vi "Close.vi"(8 "error in (no error)":errorcluster, 11 "Data in":refnum<class "Local Bus.lvclass">) -> (0 "error out":errorcluster, 3 "Data out":refnum<class "Local Bus.lvclass">)   [LabVIEW 2021, in "Local Bus.lvclass"]
uses:
  Local Bus.lvclass
  Local Bus.lvclass/Local Bus.ctl
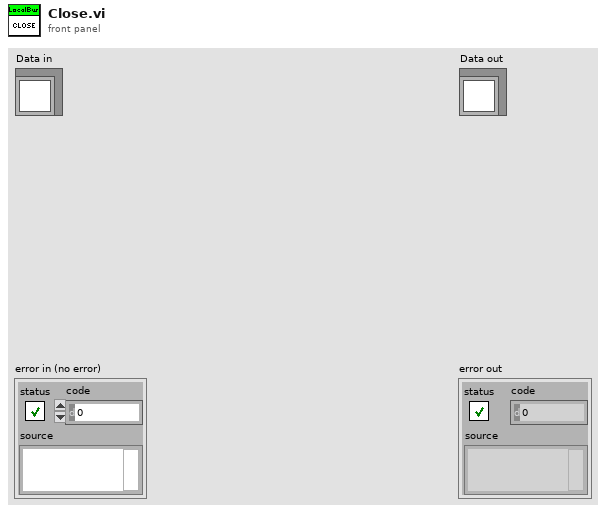
[diagram p1: front panel]
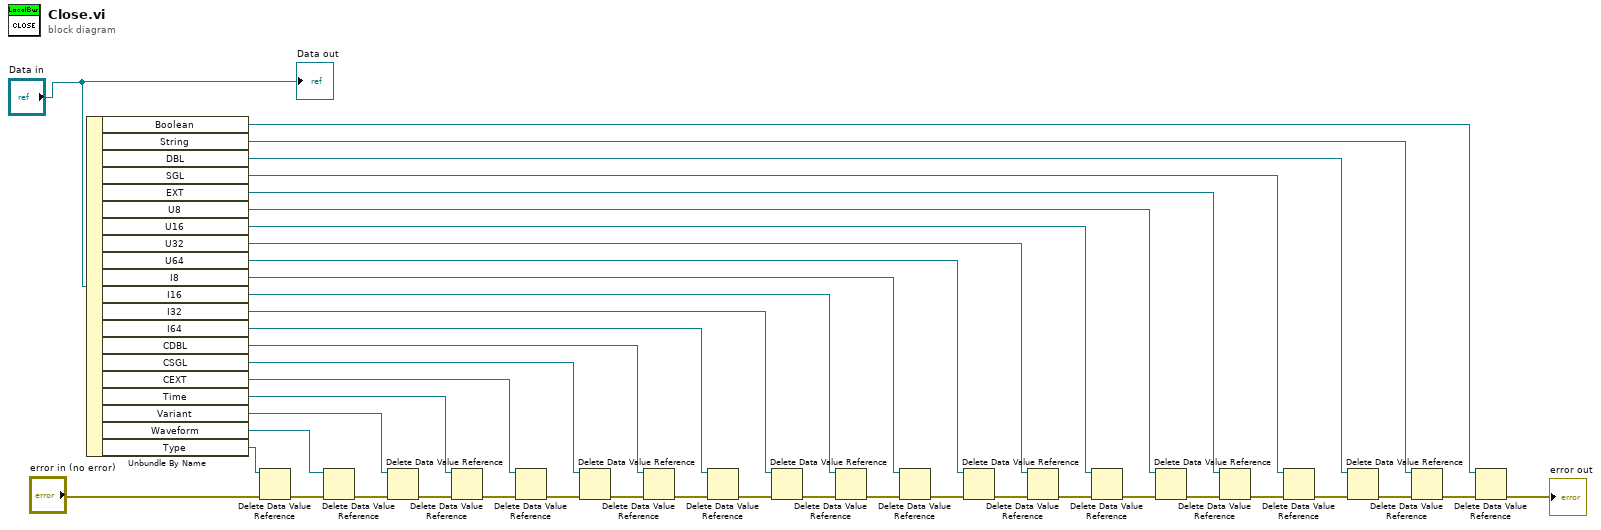
[diagram p0: block diagram]
diagram:
  n1 = Unbundle By Name("Data in") -> ("Boolean"=w4:refnum<data-value>, "String"=w5:refnum<data-value>, "DBL"=w6:refnum<data-value>, "SGL"=w7:refnum<data-value>, "EXT"=w8:refnum<data-value>, "U8"=w9:refnum<data-value>, "U16"=w10:refnum<data-value>, "U32"=w11:refnum<data-value>, "U64"=w12:refnum<data-value>, "I8"=w13:refnum<data-value>, "I16"=w14:refnum<data-value>, "I32"=w15:refnum<data-value>, "I64"=w16:refnum<data-value>, "CDBL"=w17:refnum<data-value>, "CSGL"=w18:refnum<data-value>, "CEXT"=w19:refnum<data-value>, "Time"=w20:refnum<data-value>, "Variant"=w21:refnum<data-value>, "Waveform"=w22:refnum<data-value>, "Type"=w1:refnum<data-value>)
  n2 = Delete Data Value Reference(data value reference=w1, error in="error in (no error)") -> (error out=w2:errorcluster)  [unwired: 1 out]
  n3 = Delete Data Value Reference(data value reference=w22, error in=w2) -> (error out=w42:errorcluster)  [unwired: 1 out]
  n4 = Delete Data Value Reference(data value reference=w21, error in=w42) -> (error out=w41:errorcluster)  [unwired: 1 out]
  n5 = Delete Data Value Reference(data value reference=w20, error in=w41) -> (error out=w40:errorcluster)  [unwired: 1 out]
  n6 = Delete Data Value Reference(data value reference=w19, error in=w40) -> (error out=w39:errorcluster)  [unwired: 1 out]
  n7 = Delete Data Value Reference(data value reference=w18, error in=w39) -> (error out=w38:errorcluster)  [unwired: 1 out]
  n8 = Delete Data Value Reference(data value reference=w17, error in=w38) -> (error out=w37:errorcluster)  [unwired: 1 out]
  n9 = Delete Data Value Reference(data value reference=w16, error in=w37) -> (error out=w36:errorcluster)  [unwired: 1 out]
  n10 = Delete Data Value Reference(data value reference=w15, error in=w36) -> (error out=w35:errorcluster)  [unwired: 1 out]
  n11 = Delete Data Value Reference(data value reference=w14, error in=w35) -> (error out=w34:errorcluster)  [unwired: 1 out]
  n12 = Delete Data Value Reference(data value reference=w13, error in=w34) -> (error out=w33:errorcluster)  [unwired: 1 out]
  n13 = Delete Data Value Reference(data value reference=w12, error in=w33) -> (error out=w32:errorcluster)  [unwired: 1 out]
  n14 = Delete Data Value Reference(data value reference=w11, error in=w32) -> (error out=w31:errorcluster)  [unwired: 1 out]
  n15 = Delete Data Value Reference(data value reference=w10, error in=w31) -> (error out=w30:errorcluster)  [unwired: 1 out]
  n16 = Delete Data Value Reference(data value reference=w9, error in=w30) -> (error out=w29:errorcluster)  [unwired: 1 out]
  n17 = Delete Data Value Reference(data value reference=w8, error in=w29) -> (error out=w28:errorcluster)  [unwired: 1 out]
  n18 = Delete Data Value Reference(data value reference=w7, error in=w28) -> (error out=w25:errorcluster)  [unwired: 1 out]
  n19 = Delete Data Value Reference(data value reference=w6, error in=w25) -> (error out=w26:errorcluster)  [unwired: 1 out]
  n20 = Delete Data Value Reference(data value reference=w5, error in=w26) -> (error out=w27:errorcluster)  [unwired: 1 out]
  n21 = Delete Data Value Reference(data value reference=w4, error in=w27) -> (error out=→"error out":errorcluster)  [unwired: 1 out]
  "Data out" <- "Data in"
